vi "signal_amp_unit_FGV.vi"(8 "Error In":errorcluster, 9 "Base Unit":string, 10 "Unit (Not F)":string, 11 "Action":T1) -> (0 "Error Out":errorcluster, 2 "Base":string, 3 "Unit (Not F)":string)   [LabVIEW 2021, in "Signal.lvlib"]
doc: "This FGV is used to remeber the electircal unit (V,A,Ohm, W etc)"
uses:
  Signal.lvlib
  Tipski Definicii/Unit.ctl
panel:
  # "Input"
  # "Output"
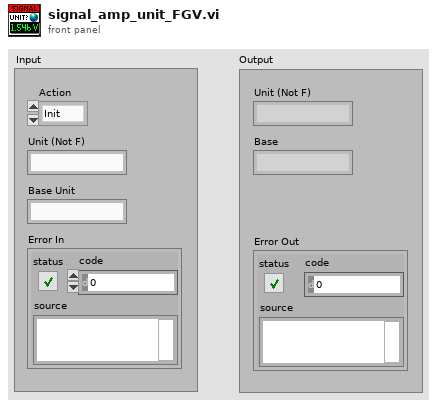
[diagram p1: front panel]
types:
  T1 = typedef "Unit.ctl" = enum16{"Init", "Add", "Read"}
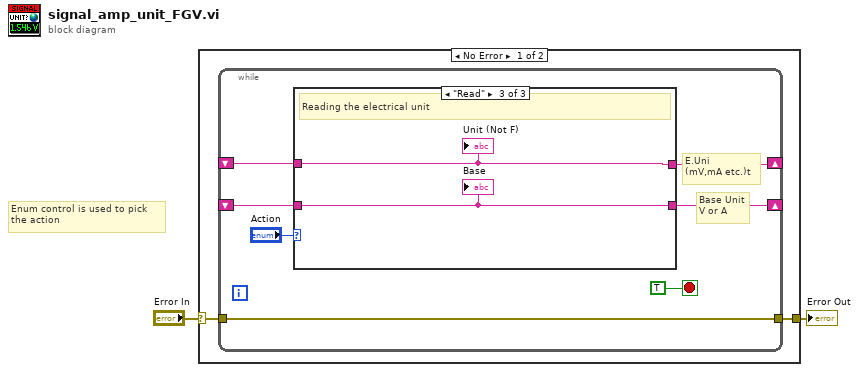
[diagram p0: block diagram]
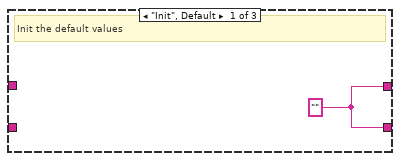
[diagram p2: hidden frame]
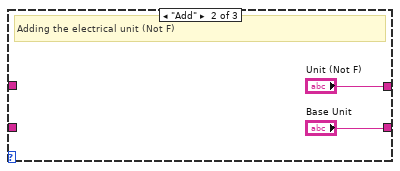
[diagram p3: hidden frame]
diagram:
  # "Enum control is used to pick \nthe action"
  n1 = case shown="No Error" "Error In" {
    selector: "Error In" -> [w4 w17]
    tunnel: [w3 w17] -> w1
    frame No Error {
      n2 = while {
        shift-right: [w9] -> _
        shift-left: _ -> [w7]
        tunnel: [w8] -> w3
        tunnel: w4 -> [w8]
        shift-right: [w6] -> _
        shift-left: _ -> [w5]
        stop <- TRUE stop-if-true
        # "Base Unit\nV or A"
        # "E.Uni\n(mV,mA etc.)t"
        n3 = case shown="\"Read\"" "Action" {
          tunnel: [w12 "Unit (Not F)" w16] -> w9
          tunnel: w7 -> [_ _ w16]
          tunnel: [w12 "Base Unit" w15] -> w6
          tunnel: w5 -> [_ _ w15]
          frame "Init", Default {
            w12 = ""
            # "Init the default values"
          }
          frame "Add" {
            # "Adding the electrical unit (Not F)"
          }
          frame "Read" {
            # "Reading the electrical unit"
            "Unit (Not F)" <- w16
            "Base" <- w15
          }
        }
      }
    }
    frame Error {
    }
  }
  "Error Out" <- w1
